vi "getTetRecChannels.vi"(6 "error in (no error)":errorcluster, 9 "shared variable refnum in":refnum<k21>="ni.var.psp://at-s1no1/AcquisitionVariables/ChannelNames") -> (0 "error out":errorcluster, 2 "TetChanNum":i32[](array[numeric]), 3 "TetNum":i32[](array[numeric]))   [LabVIEW 2010]
uses:
  <vilib>/regexp/Match Regular Expression.xnode
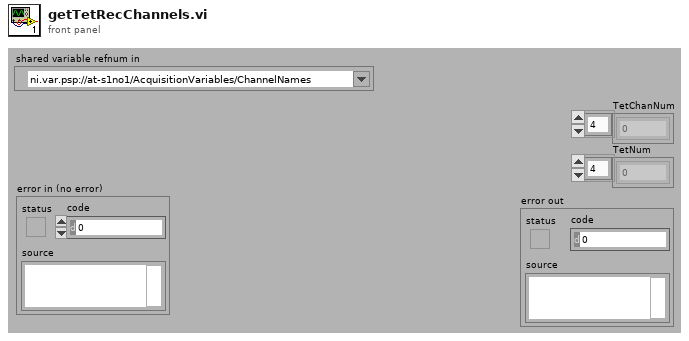
[diagram p1: front panel]
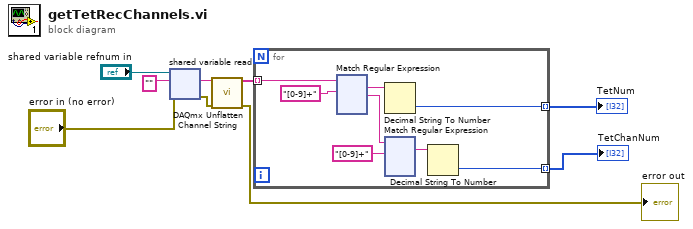
[diagram p0: block diagram]
diagram:
  n1 = shared-variable-read("shared variable refnum in", "error in (no error)", "") -> (w4:errorcluster, w7:string)  [unwired: 2 out]
  n2 = call <vilib>:"DAQmx Unflatten Channel String.vi"("names in"=w7, "error in"=w4) -> ("names out"=w6:string[], "error out"=→"error out":errorcluster)  [unwired: 12 in]
  n3 = for {
    tunnel: w6 -> [w16] mode=indexing
    tunnel: [w11] -> w2 mode=indexing
    tunnel: [w10] -> w1 mode=indexing
    n4 = xnode "Match Regular Expression"("input string"=w16, "regular expression"="[0-9]+") -> ("whole match"=w13:string, "after match"=w14:string)  [unwired: 4 in, 3 out]
    n5 = Decimal String To Number(string=w13) -> (number=w11:i32)  [unwired: 2 in, 1 out]
    n6 = xnode "Match Regular Expression"("input string"=w14, "regular expression"="[0-9]+") -> ("whole match"=w12:string)  [unwired: 4 in, 4 out]
    n7 = Decimal String To Number(string=w12) -> (number=w10:i32)  [unwired: 2 in, 1 out]
  }
  "TetChanNum" <- w1
  "TetNum" <- w2
